vi "H5Gclose.vi"(3 "group_id":i32, 9 "error in (no error)":errorcluster) -> (0 "status":i32, 6 "error out":errorcluster)   [LabVIEW 2009]
uses:
  hdf5dll.dll
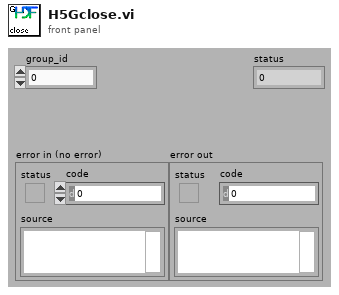
[diagram p1: front panel]
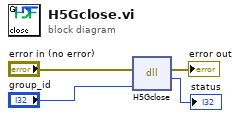
[diagram p0: block diagram]
diagram:
  n1 = dll-call lib="hdf5dll.dll" fn="H5Gclose"(error in="error in (no error)", "group_id"="group_id") -> (error out=→"error out":errorcluster, "return type"=→"status":i32)  [unwired: 3 in, 1 out]
